vi "delete_ AO config not UI to UI.vi"(8 "error in (no error)":errorcluster, 11 "AO Config":T1 {"output terminal configuration" items=["Default"=-1, "RSE"=10083, "Differential"=10106, "Pseudodifferential"=12529]}) -> (0 "error out":errorcluster, 2 "output terminal configuration":i32[](array[numeric]), 3 "AO Config (UI)":T5)   [LabVIEW 2019, in "Instrument.Lockin.lvclass"]
uses:
  Instrument.Lockin.lvclass
  Instrument.DAQ/Typedefs/AO.config(UI)-array.ctl
  Instrument.DAQ/Typedefs/AO.config(UI)-cluster.ctl
  Instrument.DAQ/Typedefs/446xAO-enum.ctl
  Instrument.DAQ/Typedefs/AO.config-array.ctl
  Instrument.DAQ/Typedefs/AO.config-cluster.ctl
  Instrument.DAQ/Typedefs/DAQType-enum.ctl
  Instrument.DAQ/Instrument.DAQ.lvclass
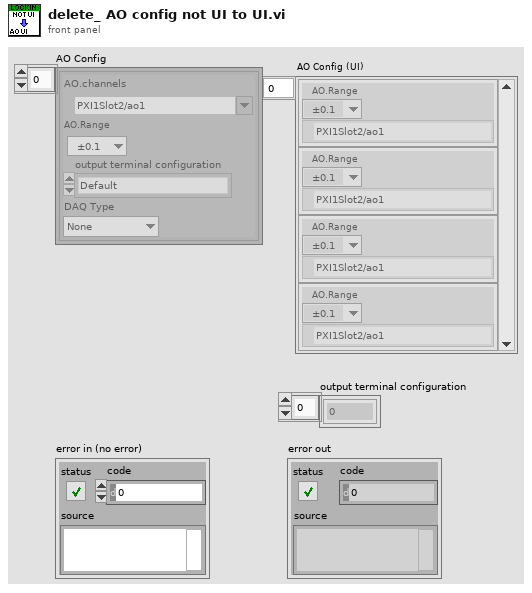
[diagram p1: front panel]
types:
  T1 = typedef "Instrument.DAQ.lvclass/AO.config-array.ctl" = T2[]
  T2 = typedef "Instrument.DAQ.lvclass/AO.config-cluster.ctl" = cluster{"AO.channels":tag, "AO.Range":T3, "output terminal configuration":i32, "DAQ Type":T4}
  T3 = typedef "Instrument.DAQ.lvclass/446xAO-enum.ctl" = enum16{"±0.1", "±1.0", "±10.0"}
  T4 = typedef "Instrument.DAQ.lvclass/DAQType-enum.ctl" = enum16{"None", "USB 4431", "PXI 446x"}
  T5 = typedef "Instrument.DAQ.lvclass/AO.config(UI)-array.ctl" = T6[]
  T6 = typedef "Instrument.DAQ.lvclass/AO.config(UI)-cluster.ctl" = cluster{"AO.Range":T3, "AO.channels":tag}
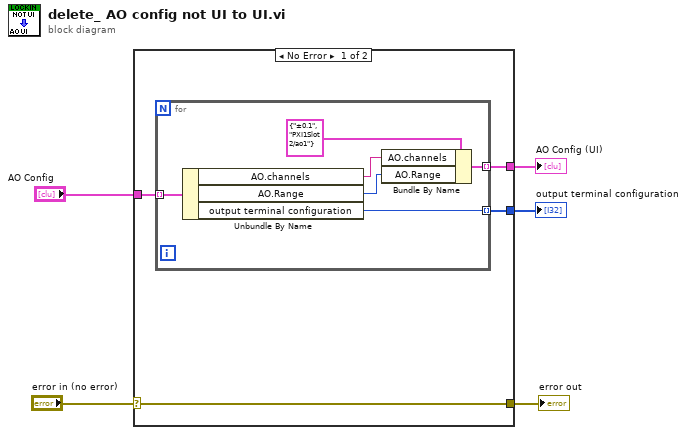
[diagram p0: block diagram]
diagram:
  n1 = case shown="No Error" "error in (no error)" {
    selector: "error in (no error)" -> [w6 w16]
    tunnel: "AO Config" -> [w9 _]
    tunnel: [w8 _] -> w4
    tunnel: [w7 _] -> w3
    tunnel: [w6 w16] -> w1
    frame No Error {
      n2 = for {
        tunnel: w9 -> [w15] mode=indexing
        tunnel: [w12] -> w8 mode=indexing
        tunnel: [w11] -> w7 mode=indexing
        n3 = Unbundle By Name(w15) -> ("AO.channels"=w14:tag, "AO.Range"=w13:T3, "output terminal configuration"=w11:i32)
        n4 = Bundle By Name(cluster=T6 {"AO.Range"=enum."±0.1", "AO.channels"="PXI1Slot2/ao1"} ("Cluster"), "AO.channels"=w14, "AO.Range"=w13) -> (w12:T6)
      }
    }
    frame Error {
    }
  }
  "AO Config (UI)" <- w4
  "output terminal configuration" <- w3
  "error out" <- w1
